vi "Throw error if blacklisted.vi"(8 "error in (no error)":errorcluster, 9 "Channel 2":string, 10 "Channel 1":string, 11 "SLSC Switch in":refnum<class "SLSC Switch.lvclass">) -> (0 "error out":errorcluster, 2 "index":i32, 3 "SLSC Switch out":refnum<class "SLSC Switch.lvclass">)   [LabVIEW 2015, in "SLSC Switch.lvclass"]
uses:
  SLSC Switch.lvclass
  Controls/Connection.ctl
  SLSC Switch.lvclass/SLSC Switch.ctl
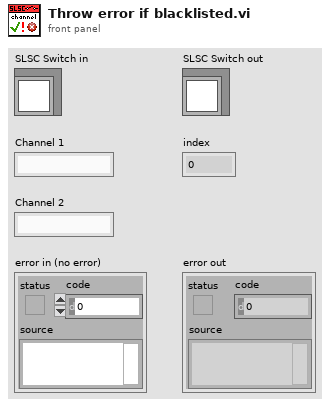
[diagram p1: front panel]
types:
  T1 = typedef "SLSC Switch.lvclass/Connection.ctl" = cluster{"channel 1":string, "channel 2":string}
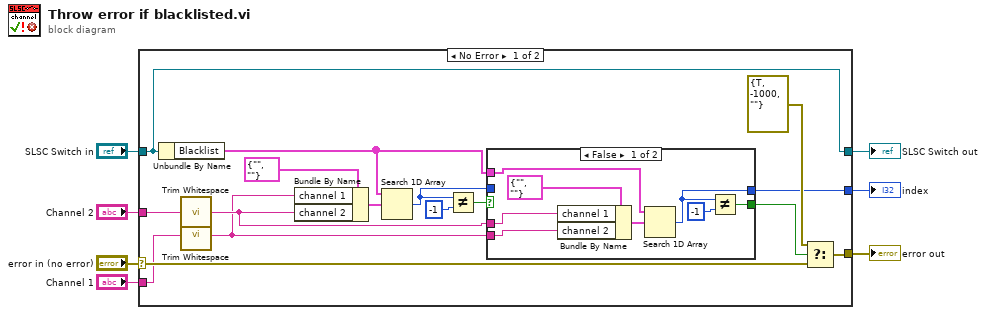
[diagram p0: block diagram]
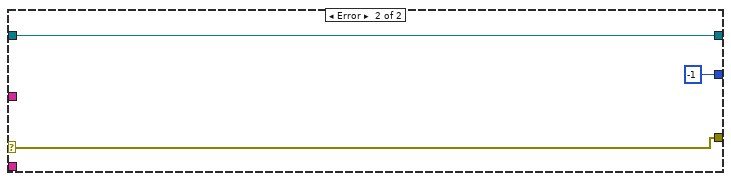
[diagram p3: hidden frame]
diagram:
  n1 = case shown="No Error" "error in (no error)" {
    selector: "error in (no error)" -> [w16 w36]
    tunnel: [w14 w36] -> w6
    tunnel: [w23 w35] -> w4
    tunnel: "SLSC Switch in" -> [w23 w35]
    tunnel: "Channel 1" -> [w9 _]
    tunnel: "Channel 2" -> [w11 _]
    tunnel: [w12 -1 ("index of element")] -> w1
    frame No Error {
      n2 = Unbundle By Name(w23) -> ("Blacklist"=w18:T1[])
      n3 = call <vilib>:"Trim Whitespace.vi"("string"=w11) -> ("trimmed string"=w10:string)  [unwired: 1 in]
      n4 = call <vilib>:"Trim Whitespace.vi"("string"=w9) -> ("trimmed string"=w8:string)  [unwired: 1 in]
      n5 = Bundle By Name(cluster=T1 {"channel 1"="", "channel 2"=""} ("connections"), "channel 1"=w8, "channel 2"=w10) -> (w20:T1)
      n6 = Search 1D Array(1D array=w18, element=w20) -> (index of element=w13:i32)  [unwired: 1 in]
      n7 = Not Equal?(x=w13, y=-1) -> (x != y?=w19:bool)
      n8 = case shown="False" w19 {
        selector: w19 -> [_ w33]
        tunnel: [w25 w33] -> w17
        tunnel: w18 -> [w28 _]
        tunnel: w10 -> [w27 _]
        tunnel: w8 -> [w26 _]
        tunnel: w13 -> [_ w32]
        tunnel: [w24 w32] -> w12
        frame False {
          n9 = Bundle By Name(cluster=T1 {"channel 1"="", "channel 2"=""} ("connections"), "channel 1"=w27, "channel 2"=w26) -> (w31:T1)
          n10 = Search 1D Array(1D array=w28, element=w31) -> (index of element=w24:i32)  [unwired: 1 in]
          n11 = Not Equal?(x=w24, y=-1) -> (x != y?=w25:bool)
        }
        frame True {
        }
      }
      n12 = Select(t=errorcluster {"status"=TRUE, "code"=-1000, "source"=""}, s=w17, f=w16) -> (s? t:f=w14:errorcluster)
    }
    frame Error {
    }
  }
  "error out" <- w6
  "SLSC Switch out" <- w4
  "index" <- w1
